vi "Close.vi"(8 "error in (no error)":errorcluster, 11 "PWM CFG in":refnum<class "PWM CFG.lvclass">) -> (0 "error out":errorcluster, 3 "PWM CFG out":refnum<class "PWM CFG.lvclass">)   [LabVIEW 2023, in "DIO Simulated.lvlib" / "PWM CFG.lvclass"]
uses:
  PWM CFG.lvclass
  PWM CFG.lvclass/PWM CFG.ctl
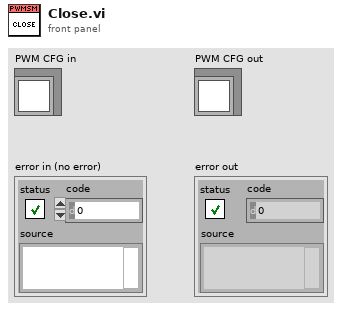
[diagram p1: front panel]
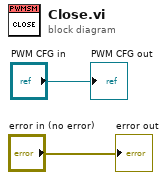
[diagram p0: block diagram]
diagram:
  "error out" <- "error in (no error)"
  "PWM CFG out" <- "PWM CFG in"
